vi "FTW-Subscriber-Destroy.vi"(0 "FTW Subscriber":refnum<data-value>, 11 "error in":errorcluster) -> (15 "error out":errorcluster)   [LabVIEW 2014]
uses:
  core/FTW-Subscriber-Core-Type.ctl
panel:
  # "Inputs"
  # "Outputs"
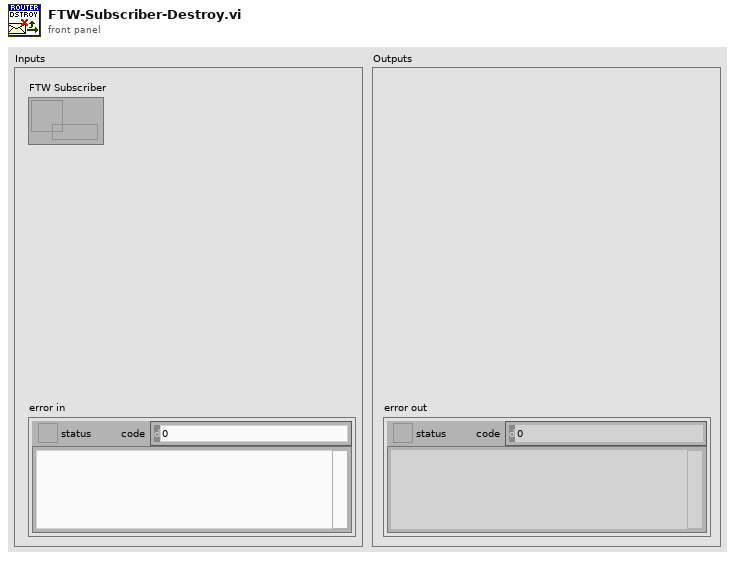
[diagram p1: front panel]
types:
  T1 = typedef "FTW-Subscriber-Core-Type.ctl" = cluster{"Socket":i64, "SubscriptionEvent":refnum<user-event>}
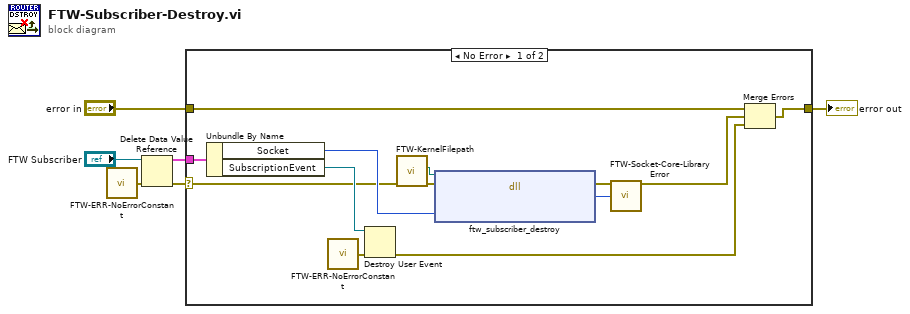
[diagram p0: block diagram]
diagram:
  n1 = call "FTW-ERR-NoErrorConstant.vi"() -> ("no error"=w1:errorcluster)
  n2 = Delete Data Value Reference(data value reference="FTW Subscriber", error in=w1) -> (data value=w3:T1, error out=w2:errorcluster)
  n3 = case shown="No Error" w2 {
    selector: w2 -> [w9 _]
    tunnel: [w19 w20] -> w6
    tunnel: "error in" -> [w17 w20]
    tunnel: w3 -> [w13 _]
    frame No Error {
      n4 = Unbundle By Name(w13) -> ("Socket"=w16:i64, "SubscriptionEvent"=w15:refnum<user-event>)
      n5 = call "FTW-ERR-NoErrorConstant.vi"() -> ("no error"=w14:errorcluster)
      n6 = Destroy User Event(user event=w15, error in=w14) -> (error out=w12:errorcluster)
      n7 = call "FTW-KernelFilepath.vi"("error in"=w9) -> ("error out"=w8:errorcluster, "Library Filepath"=w7:path)  [unwired: 8 in, 1 out]
      n8 = dll-call lib="?" fn="ftw_subscriber_destroy"(path in=w7, error in=w8, "Socket Handle"=w16) -> (error out=w11:errorcluster, "Return Value"=w10:i64)  [unwired: 2 in, 1 out]
      n9 = call "FTW-Socket-Core-LibraryError.vi"("error in"=w11, "Return Value"=w10) -> ("error out"=w18:errorcluster)  [unwired: 13 in]
      n10 = Merge Errors(w17, w18, w12) -> (w19:errorcluster)
    }
    frame Error {
    }
  }
  "error out" <- w6
